vi "YFM1.vi"() -> ()   [LabVIEW 2017]
uses:
  <vilib>/DAQmx/write.llb/DAQmx Write (Analog DBL 1Chan 1Samp).vi
  <vilib>/DAQmx/read.llb/DAQmx Read (Analog 1D DBL 1Chan NSamp).vi
  <vilib>/DAQmx/create/channels.llb/DAQmx Create Channel (AO-Voltage-Basic).vi
  <vilib>/DAQmx/create/channels.llb/DAQmx Create Channel (AI-Voltage-Basic).vi
  <vilib>/DAQmx/configure/timing.llb/DAQmx Timing (Sample Clock).vi
  <vilib>/DAQmx/miscellaneous.llb/DAQmx Fill In Error Info.vi
  <vilib>/measure/NI_MABase.lvlib
  <vilib>/Analysis/NI_AALPro.lvlib
panel:
  out "Array":dbl[](array[numeric])
  out "Vg Array":dbl[](array[numeric])
  out "Rct":dbl
  out "theta":cluster{"X":dbl, "Y":dbl}[](graph)
  out "YFM":cluster{"Y":dbl[], dbl[]}(graph)
  out "gm":cluster{"dX/dt":dbl[], "Y":dbl[]}(graph)
  out "error out 3":errorcluster={"status"=TRUE, "code"=-200099, "source"="DAQmx Create Channel (AO-Voltage-Basic).vi:1870002<append>\n<B>Task Name: </B>_unnamedTask<0>"}
  in  "error in 3":errorcluster
  out "transfer characteristic":cluster{"Y":dbl[], "Y":dbl[]}(graph)
  in  "Vd":dbl
  in  "Vd channels":tag="Dev3/ao1"
  out "error out 2":errorcluster
  in  "error in 2":errorcluster
  out "error out":errorcluster={"status"=TRUE, "code"=-200477, "source"="YFM.vi<append>\n<B>Task Name: </B>_unnamedTask<1>"}
  in  "Id channels":tag="Dev9/ai0"
  out "# of step":dbl=nan
  in  "Step":dbl=0.1
  in  "Stop (V)":dbl=2.0
  in  "Start (V)":dbl=1.0
  in  "error in":errorcluster
  in  "Vg channels":tag="Dev3/ao0"
  # "Vg"
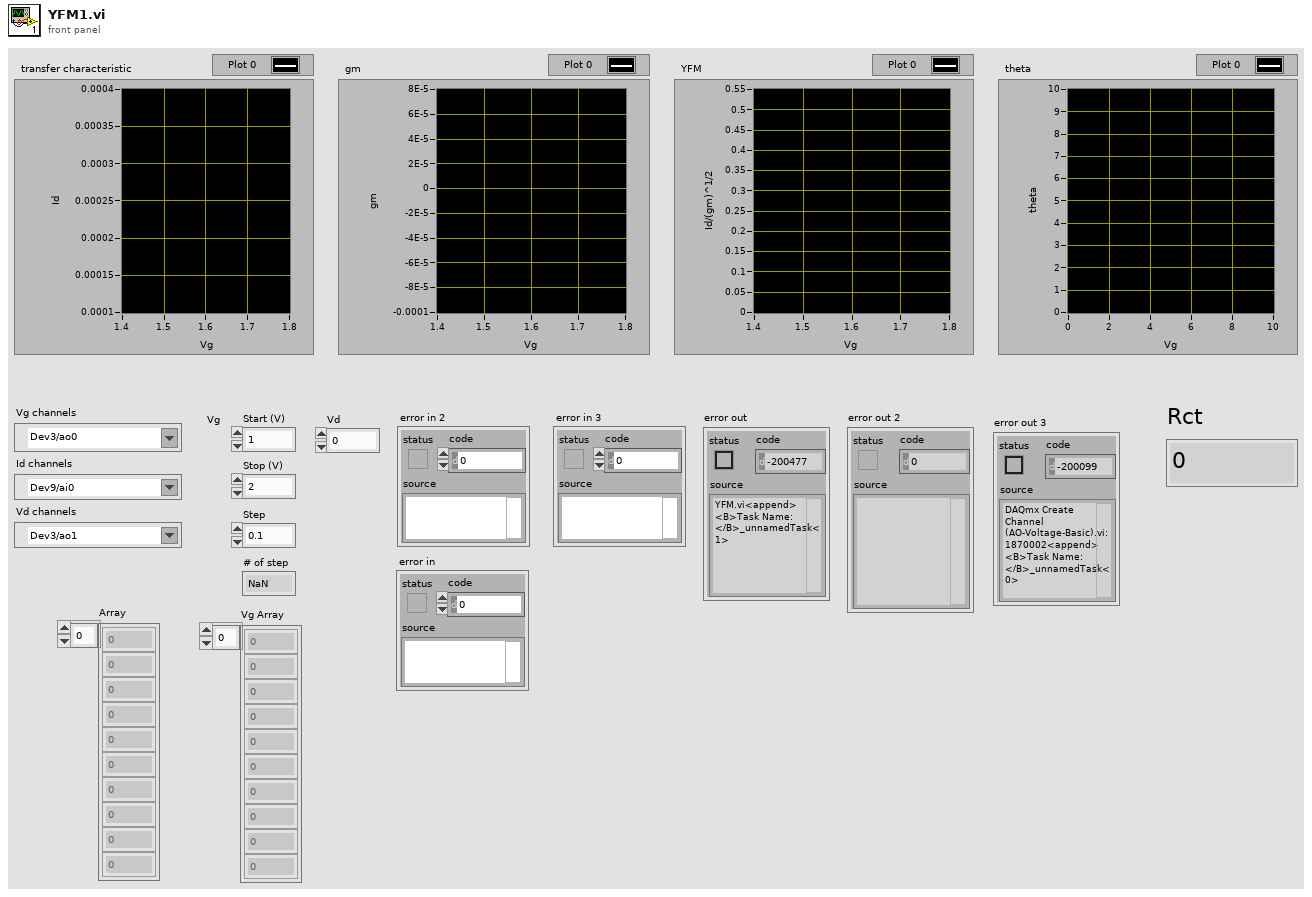
[diagram p1: front panel]
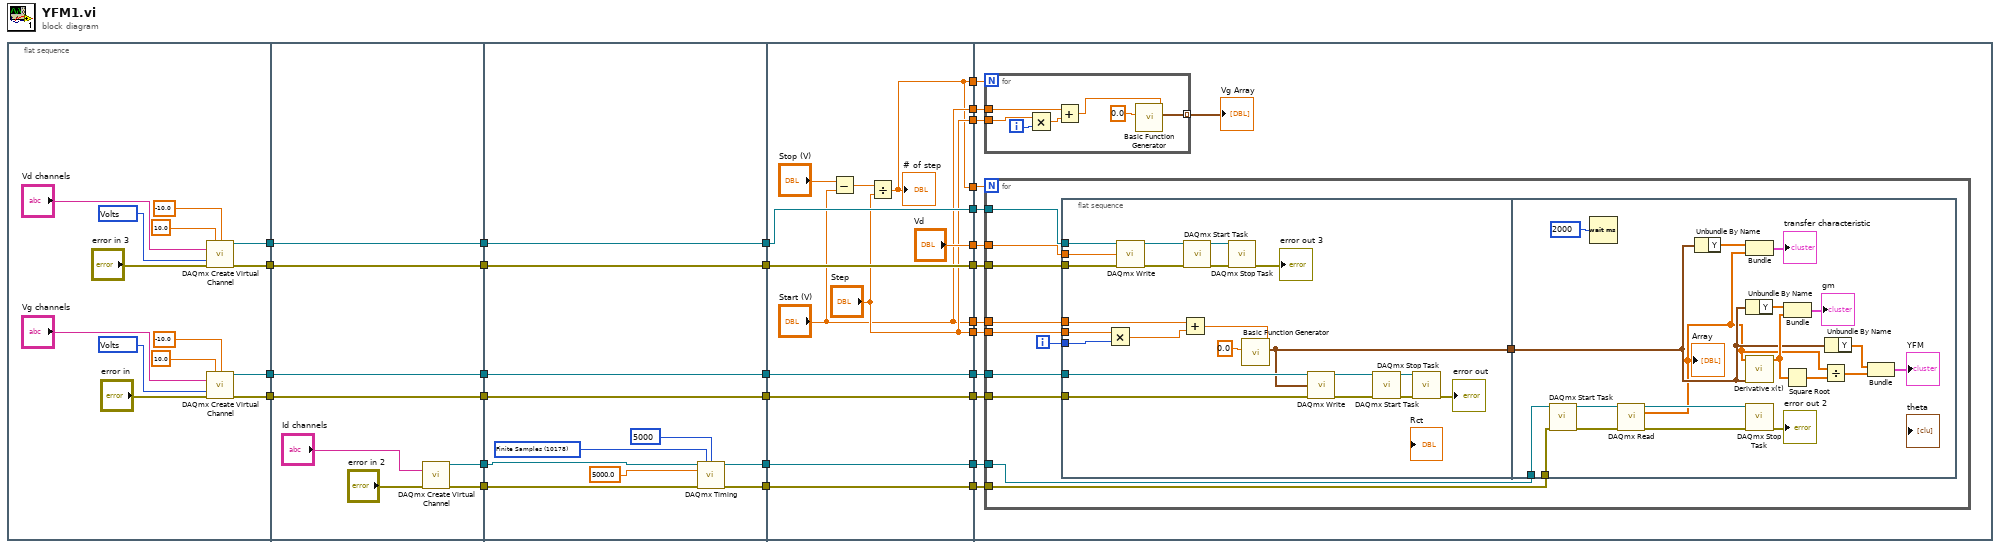
[diagram p0: block diagram]
diagram:
  n1 = flat-sequence {
    tunnel: [w38] -> w18
    tunnel: [w37] -> w16
    tunnel: [w32] -> w8
    tunnel: [w31] -> w4
    tunnel: w18 -> [w51]
    tunnel: [w51] -> w17
    tunnel: w16 -> [w50]
    tunnel: [w50] -> w15
    tunnel: [w47] -> w14
    tunnel: [w46] -> w13
    tunnel: [w45] -> w9
    tunnel: w8 -> [w45]
    tunnel: [w44] -> w5
    tunnel: w4 -> [w44]
    tunnel: w17 -> [w62]
    tunnel: w15 -> [w61]
    tunnel: w14 -> [w60]
    tunnel: w13 -> [w56]
    tunnel: [w62] -> w29
    tunnel: [w61] -> w28
    tunnel: [w55] -> w27
    tunnel: [w54] -> w26
    tunnel: [w53] -> w10
    tunnel: w9 -> [w53]
    tunnel: [w52] -> w6
    tunnel: w5 -> [w52]
    tunnel: w29 -> [w74]
    tunnel: w28 -> [w73]
    tunnel: w27 -> [w72]
    tunnel: w26 -> [w71]
    tunnel: [w74] -> w25
    tunnel: [w73] -> w24
    tunnel: [w72] -> w23
    tunnel: [w71] -> w22
    tunnel: ["Step"] -> w21
    tunnel: ["Start (V)"] -> w20
    tunnel: [w63] -> w19
    tunnel: ["Vd"] -> w12
    tunnel: [w67] -> w11
    tunnel: w10 -> [w67]
    tunnel: [w66] -> w7
    tunnel: w6 -> [w66]
    tunnel: ["Step"] -> w3
    tunnel: ["Start (V)"] -> w2
    tunnel: [w63] -> w1
    tunnel: w25 -> [w86]
    tunnel: w24 -> [w85]
    tunnel: w23 -> [w83]
    tunnel: w22 -> [w82]
    tunnel: w21 -> [w88]
    tunnel: w20 -> [w87]
    tunnel: w19 -> [w84]
    tunnel: w12 -> [w81]
    tunnel: w11 -> [w80]
    tunnel: w7 -> [w79]
    tunnel: w3 -> [w78]
    tunnel: w2 -> [w77]
    tunnel: w1 -> [w76]
    frame #0 {
      w34 = 10348 items=["Volts"=10348, "From Custom Scale"=10065] ("units")
      w39 = 10348 items=["Volts"=10348, "From Custom Scale"=10065] ("units")
      n2 = call-poly <vilib>:"DAQmx Create Virtual Channel.vi"("maximum value"=10.0, "minimum value"=-10.0, "physical channels"="Vd channels", "units"=w34, "error in"="error in 3") -> ("task out"=w32:refnum<k21>, "error out"=w31:errorcluster)  [unwired: 9 in]
      n3 = call-poly <vilib>:"DAQmx Create Virtual Channel.vi"("maximum value"=10.0, "minimum value"=-10.0, "physical channels"="Vg channels", "units"=w39, "error in"="error in") -> ("task out"=w38:refnum<k21>, "error out"=w37:errorcluster)  [unwired: 9 in]
    }
    frame #1 {
      n4 = call-poly <vilib>:"DAQmx Create Virtual Channel.vi"("physical channels"="Id channels", "error in"="error in 2") -> ("task out"=w47:refnum<k21>, "error out"=w46:errorcluster)  [unwired: 12 in]
    }
    frame #2 {
      w59 = 10178 items=["Finite Samples"=10178, "Continuous Samples"=10123, "Hardware Timed Single Point"=12522] ("sample mode")
      n5 = call-poly <vilib>:"DAQmx Timing.vi"("task/channels in"=w60, "sample mode"=w59, "samples per channel"=5000, "rate"=5000.0, "error in"=w56) -> ("task out"=w55:refnum<k21>, "error out"=w54:errorcluster)  [unwired: 9 in]
    }
    frame #3 {
      n6 = Subtract(x="Stop (V)", y="Start (V)") -> (x-y=w70:dbl)
      n7 = Divide(x=w70, y="Step") -> (x/y=w63:dbl)
      "# of step" <- w63
    }
    frame #4 {
      n8 = for {
        N: w76 -> [_]
        tunnel: w78 -> [w93]
        tunnel: w77 -> [w92]
        tunnel: [w89] -> w75 mode=indexing
        i -> [w94]
        n9 = Multiply(x=w93, y=w94) -> (x*y=w95:dbl)
        n10 = Add(x=w92, y=w95) -> (x+y=w91:dbl)
        n11 = call <vilib>:"Basic Function Generator.vi"("offset"=w91, "amplitude"=0.0) -> ("signal out"=w89:waveform(dbl))  [unwired: 7 in, 2 out]
      }
      "Vg Array" <- w75
      n12 = for {
        N: w84 -> [_]
        tunnel: w88 -> [w105]
        tunnel: w87 -> [w104]
        tunnel: w86 -> [w103]
        tunnel: w85 -> [w96]
        tunnel: w83 -> [w102]
        tunnel: w82 -> [w101]
        tunnel: w81 -> [w100]
        tunnel: w80 -> [w99]
        tunnel: w79 -> [w98]
        i -> [w106]
        n13 = flat-sequence {
          tunnel: w106 -> [w124]
          tunnel: w105 -> [w123]
          tunnel: w104 -> [w122]
          tunnel: w103 -> [w121]
          tunnel: w100 -> [w120]
          tunnel: w99 -> [w117]
          tunnel: w98 -> [w116]
          tunnel: [w107] -> w97
          tunnel: w96 -> [w109]
          tunnel: w102 -> [w145]
          tunnel: w101 -> [w144]
          tunnel: w97 -> [w132]
          frame #0 {
            n14 = Multiply(x=w123, y=w124) -> (x*y=w128:dbl)
            n15 = call-poly <vilib>:"DAQmx Write.vi"("task/channels in"=w117, "data"=w120, "error in"=w116) -> ("task out"=w119:refnum<k21>, "error out"=w115:errorcluster)  [unwired: 10 in, 1 out]
            n16 = Add(x=w122, y=w128) -> (x+y=w127:dbl)
            n17 = call <vilib>:"DAQmx Start Task.vi"("task/channels in"=w119, "error in"=w115) -> ("task out"=w118:refnum<k21>, "error out"=w114:errorcluster)  [unwired: 12 in]
            n18 = call <vilib>:"DAQmx Stop Task.vi"("task/channels in"=w118, "error in"=w114) -> ("error out"=→"error out 3":errorcluster)  [unwired: 12 in, 1 out]
            n19 = call <vilib>:"Basic Function Generator.vi"("offset"=w127, "amplitude"=0.0) -> ("signal out"=w107:waveform(dbl))  [unwired: 7 in, 2 out]
            n20 = call-poly <vilib>:"DAQmx Write.vi"("task/channels in"=w121, "data"=w107, "error in"=w109) -> ("task out"=w126:refnum<k21>, "error out"=w125:errorcluster)  [unwired: 10 in, 1 out]
            n21 = call <vilib>:"DAQmx Start Task.vi"("task/channels in"=w126, "error in"=w125) -> ("task out"=w112:refnum<k21>, "error out"=w111:errorcluster)  [unwired: 12 in]
            n22 = call <vilib>:"DAQmx Stop Task.vi"("task/channels in"=w112, "error in"=w111) -> ("error out"=→"error out":errorcluster)  [unwired: 12 in, 1 out]
          }
          frame #1 {
            n23 = call <vilib>:"DAQmx Start Task.vi"("task/channels in"=w145, "error in"=w144) -> ("task out"=w147:refnum<k21>, "error out"=w146:errorcluster)  [unwired: 12 in]
            n24 = Wait (ms)(milliseconds to wait=u32 2000) -> ()  [unwired: 1 out]
            n25 = call-poly <vilib>:"DAQmx Read.vi"("task/channels in"=w147, "error in"=w146) -> ("task out"=w142:refnum<k21>, "data"=w129:dbl[], "error out"=w141:errorcluster)  [unwired: 11 in]
            "Array" <- w129
            n26 = Unbundle By Name(w132) -> ("Y"=w130:dbl[])
            n27 = Bundle("Y"=w130, "data"=w129) -> (→"transfer characteristic":cluster{"Y":dbl[], "data":dbl[]})  [unwired: 1 in]
            n28 = Unbundle By Name(w132) -> ("Y"=w138:dbl[])
            n29 = call <vilib>:"Derivative x(t).vi"("dt"=w132, "X"=w129) -> ("dX/dt"=w137:dbl[])  [unwired: 8 in, 1 out]
            n30 = call <vilib>:"DAQmx Stop Task.vi"("task/channels in"=w142, "error in"=w141) -> ("error out"=→"error out 2":errorcluster)  [unwired: 12 in, 1 out]
            n31 = Square Root(x=w137) -> (sqrt(x)=w136:dbl[])
            n32 = Bundle("Y"=w138, "dX/dt"=w137) -> (→"gm":cluster{"Y":dbl[], "dX/dt":dbl[]})  [unwired: 1 in]
            n33 = Divide(x=w129, y=w136) -> (x/y=w135:dbl[])
            n34 = Unbundle By Name(w132) -> ("Y"=w131:dbl[])
            n35 = Bundle("Y"=w131, w135) -> (→"YFM":cluster{"Y":dbl[], dbl[]})  [unwired: 1 in]
          }
        }
      }
    }
  }
